vi "GenerateProjectDocumentation--function.vi"(8 "error in":errorcluster, 11 "Antidoc Args":T1={"ProjectPath"=path "C:/Users/PaulONeill/SCC/Orion/LabVIEW/Source/App/Orion.lvproj", "ReportDir"=path "C:/Users/PaulONeill/SCC/Orion/LabVIEW/Antidoc-Output", "ReportFile"="Orion-Report", "ReportTitle"="Orion Architecture Report", "ReportAuthor"="Paul O'Neill", "Commit"="ehsnkwe23", "Date"="today", "Tag"="1.1.1"}) -> (0 "error out":errorcluster, 2 "Generation Details":string, 3 "Generated File":path)   [LabVIEW 2020, in "CICD.lvlib"]
uses:
  CICD.lvlib
  AntidocArgs2--cluster.ctl
  <vilib>/Wovalab/AntiDoc/Doc/Author Info--cluster.ctl
  <vilib>/Wovalab/AntiDoc/Document Type/Document/Document Type.lvclass/Document Type.ctl
  <vilib>/Wovalab/AntiDoc/Doc/Doc.lvclass/Doc.ctl
  <vilib>/Wovalab/AsciiDoc for LabVIEW/Toolchain/Output Format--enum.ctl
  <vilib>/Wovalab/AntiDoc/Doc/Write Document File Name.vi
  <vilib>/Wovalab/AntiDoc/Document Type/Document/Write Config.vi
  <vilib>/Wovalab/AntiDoc/Document Type/Add-ons/LabVIEW Project/Lv Proj Config/Lv Proj Config.lvclass
  C:/Program Files/National Instruments/LabVIEW 2020/vi.lib/Wovalab/AntiDoc/Document Type/Config/Config.lvclass
  <vilib>/Utility/error.llb/Error Cluster From Error Code.vi
  <vilib>/Wovalab/AntiDoc/Doc/Write Documentation Folder.vi
  <vilib>/Wovalab/AntiDoc/Document Type/Config/Config.lvclass
  <vilib>/Wovalab/AntiDoc/Document Type/Document/Document Type.lvclass
  <vilib>/Wovalab/AntiDoc/Doc/Doc.lvclass
  <vilib>/Wovalab/AsciiDoc for LabVIEW/Wovalab_lib_AsciiDoctor.lvlib
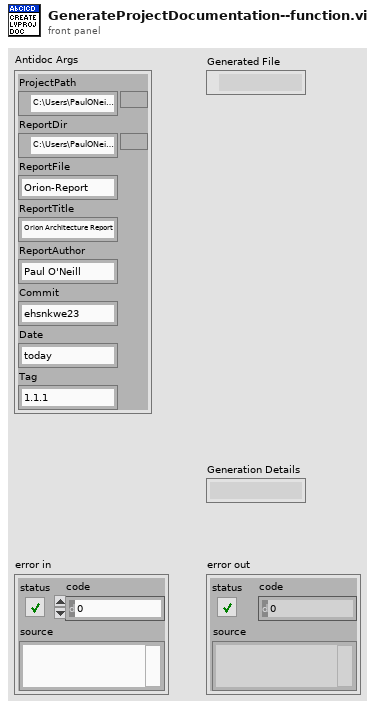
[diagram p1: front panel]
types:
  T1 = typedef "CICD.lvlib/AntidocArgs2--cluster.ctl" = cluster{"ProjectPath":path, "ReportDir":path, "ReportFile":string, "ReportTitle":string, "ReportAuthor":string, "Commit":string, "Date":string, "Tag":string}
  T2 = typedef "AntiDoc.lvlib/Doc.lvclass/Author Info--cluster.ctl" = cluster{"Name":string, "Email":string}
  T3 = typedef "Wovalab_lib_AsciiDoctor.lvlib/Output Format--enum.ctl" = enum16{"HTML5", "PDF"}
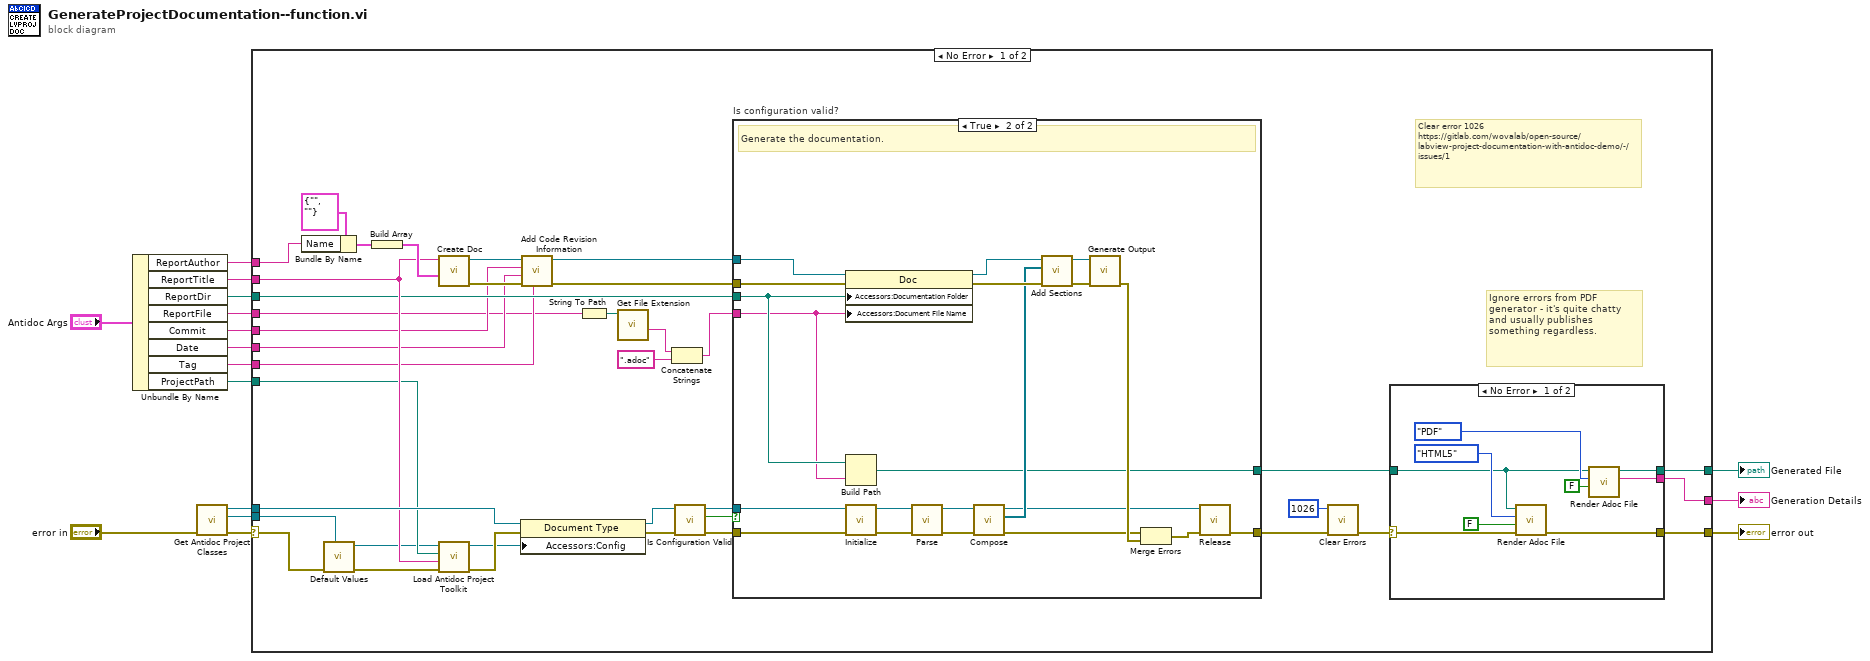
[diagram p0: block diagram]
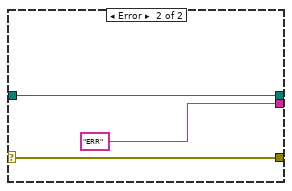
[diagram p2: hidden frame]
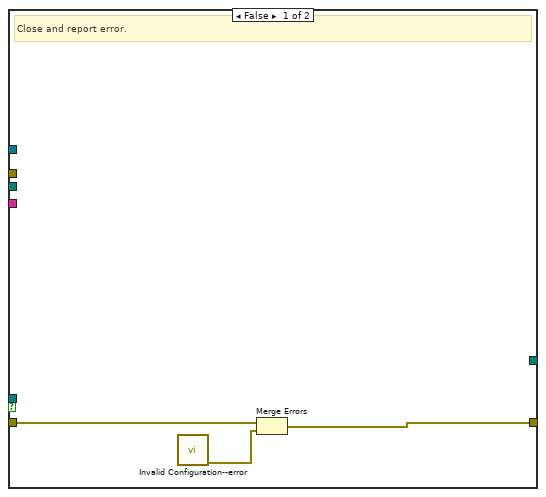
[diagram p3: hidden frame]
diagram:
  n1 = Unbundle By Name("Antidoc Args") -> ("ReportAuthor"=w7:string, "ReportTitle"=w6:string, "ReportDir"=w10:path, "ReportFile"=w9:string, "Commit"=w5:string, "Date"=w4:string, "Tag"=w3:string, "ProjectPath"=w8:path)
  n2 = call "Get Antidoc Project Classes.vi"("error in (no error)"="error in") -> ("error out"=w15:errorcluster, "Config"=w12:refnum<class "Config.lvclass">, "Document Type out"=w13:refnum<class "Document Type.lvclass">)  [unwired: 8 in]
  n3 = case shown="No Error" w15 {
    selector: w15 -> [w26 w91]
    tunnel: w13 -> [w48 _]
    tunnel: [w21 w91] -> w14
    tunnel: w12 -> [w23 _]
    tunnel: w6 -> [w41 _]
    tunnel: w7 -> [w40 _]
    tunnel: w10 -> [w39 _]
    tunnel: w9 -> [w27 _]
    tunnel: w8 -> [w35 _]
    tunnel: w5 -> [w38 _]
    tunnel: w4 -> [w37 _]
    tunnel: w3 -> [w36 _]
    tunnel: [w20 _] -> w2
    tunnel: [w19 _] -> w1
    frame No Error {
      # "Ignore errors from PDF generator - it's quite chatty and usually publishes something regardless."
      # "Clear error 1026\nhttps://gitlab.com/wovalab/open-source/labview-project-documentation-with-antidoc-demo/-/issues/1"
      n4 = Bundle By Name(cluster=T2 {"Name"="", "Email"=""} ("Author Info"), "Name"=w40) -> (w44:T2)
      n5 = call-dynamic "Default Values.vi"("Type"=w23, "error in (no error)"=w26) -> ("error out"=w25:errorcluster, "Config out"=w24:refnum<class "Config.lvclass">)  [unwired: 8 in]
      n6 = Build Array(w44) -> (w43:T2[])
      n7 = call <vilib>:"Create Doc.vi"("Authors"=w43, "Title"=w41) -> ("error out"=w54:errorcluster, "Doc out"=w47:refnum<class "Doc.lvclass">)  [unwired: 8 in]
      n8 = call "Load Antidoc Project Toolkit.vi"("error in"=w25, "Document Title"=w41, "Project Path"=w35, "Config"=w24) -> ("error out"=w51:errorcluster, "Config out"=w42:refnum<class "Lv Proj Config.lvclass">)  [unwired: 6 in]
      n9 = property class="Document Type"(reference=w48, error in=w51, "Accessors:Config"=w42) -> (reference out=w34:refnum<class "Document Type.lvclass">, error out=w52:errorcluster)
      n10 = call <vilib>:"Add Code Revision Information.vi"("Revision Info.Tag"=w36, "error in"=w54, "Revision Info.Date"=w37, "Revision Info.Commit"=w38, "Doc in"=w47) -> ("error out"=w53:errorcluster, "Doc out"=w46:refnum<class "Doc.lvclass">)  [unwired: 5 in]
      n11 = String To Path(string=w27) -> (path=w31:path)
      n12 = call <vilib>:"Get File Extension.vi"("file"=w31) -> ("filename without extension"=w30:string)  [unwired: 6 in, 4 out]
      n13 = Concatenate Strings(w30, ".adoc" ("string")) -> (w28:string)
      n14 = call-dynamic "Is Configuration Valid.vi"("error in"=w52, "Document in"=w34) -> ("error out"=w50:errorcluster, "Valid?"=w32:bool, "Document out"=w33:refnum<class "Document Type.lvclass">)  [unwired: 6 in, 1 out]
      n15 = case "Is configuration valid?" shown="True" w32 {
        tunnel: w46 -> [_ w85]
        tunnel: w53 -> [_ w89]
        tunnel: w39 -> [_ w81]
        tunnel: w50 -> [w69 w87]
        tunnel: w33 -> [_ w82]
        tunnel: [w68 w77] -> w49
        tunnel: w28 -> [_ w80]
        tunnel: [_ w76] -> w17
        frame False {
          # "Close and report error."
          n16 = call "Invalid Configuration--error.vi"() -> ("error out"=w67:errorcluster)  [unwired: 11 in]
          n17 = Merge Errors(w69, w67) -> (w68:errorcluster)
        }
        frame True {
          # "Generate the documentation."
          n18 = property class="Doc"(reference=w85, error in=w89, "Accessors:Documentation Folder"=w81, "Accessors:Document File Name"=w80) -> (reference out=w84:refnum<class "Doc.lvclass">, error out=w88:errorcluster)
          n19 = Build Path(base path=w81, name or relative path=w80) -> (appended path=w76:path)
          n20 = call-dynamic "Initialize.vi"("error in (no error)"=w87, "Document in"=w82) -> ("error out"=w75:errorcluster, "Document out"=w71:refnum<class "Document Type.lvclass">)  [unwired: 8 in]
          n21 = call-dynamic "Parse.vi"("error in (no error)"=w75, "Document in"=w71) -> ("error out"=w74:errorcluster, "Document out"=w72:refnum<class "Document Type.lvclass">)  [unwired: 8 in]
          n22 = call-dynamic "Compose.vi"("error in (no error)"=w74, "Document in"=w72) -> ("error out"=w73:errorcluster, "Sections"=w83:refnum<class "Section.lvclass">[], "Document out"=w70:refnum<class "Document Type.lvclass">)  [unwired: 7 in]
          n23 = call <vilib>:"Add Sections.vi"("error in (no error)"=w88, "Sections"=w83, "Doc in"=w84) -> ("error out"=w90:errorcluster, "Doc out"=w86:refnum<class "Doc.lvclass">)  [unwired: 7 in]
          n24 = call <vilib>:"Generate Output.vi"("error in"=w90, "Doc in"=w86) -> ("error out"=w78:errorcluster)  [unwired: 8 in, 1 out]
          n25 = Merge Errors(w73, w78) -> (w79:errorcluster)
          n26 = call-dynamic "Release.vi"("error in (no error)"=w79, "Document in"=w70) -> ("error out"=w77:errorcluster)  [unwired: 9 in]
        }
      }
      n27 = call <vilib>:"Clear Errors.vi"("error in (no error)"=w49, "specific error code to clear (0: all)"=1026) -> ("error out"=w18:errorcluster)  [unwired: 4 in, 1 out]
      n28 = case shown="No Error" w18 {
        selector: w18 -> [w61 w66]
        tunnel: [w55 w66] -> w21
        tunnel: [w60 w64] -> w20
        tunnel: [w59 "ERR" ("Generation Details")] -> w19
        tunnel: w17 -> [w56 w64]
        frame No Error {
          n29 = call <vilib>:"Render Adoc File.vi"("error in"=w61, "Open Generated Document"=FALSE, "Output Format"=Output_Format--enum."HTML5", "Adoc File Path"=w56) -> ("error out"=w55:errorcluster)  [unwired: 5 in, 2 out]
          n30 = call <vilib>:"Render Adoc File.vi"("Open Generated Document"=FALSE, "Output Format"=Output_Format--enum."PDF", "Adoc File Path"=w56) -> ("Generation Details"=w59:string, "Generated File"=w60:path)  [unwired: 6 in, 1 out]
        }
        frame Error {
        }
      }
    }
    frame Error {
    }
  }
  "error out" <- w14
  "Generated File" <- w2
  "Generation Details" <- w1
